vi "WriteData.vi"(6 "TransmissionType":T1, 8 "error in (no error)":errorcluster, 10 "Command":string, 11 "ControlState in":T2 {"ChainMask" format="0x%02x"}) -> (0 "error out":errorcluster, 1 "Data Written?":bool, 2 "return count":u32, 3 "ControlState out":T2 {"ChainMask" format="0x%02x"})   [LabVIEW 2020, in "ArduinoSerialBling.lvlib"]
uses:
  ArduinoSerialBling.lvlib
  ControlState.ctl
  ChainState.ctl
  TransmissionType.ctl
  <vilib>/Instr/_visa.llb/VISA Flush IO Buffer Mask.ctl
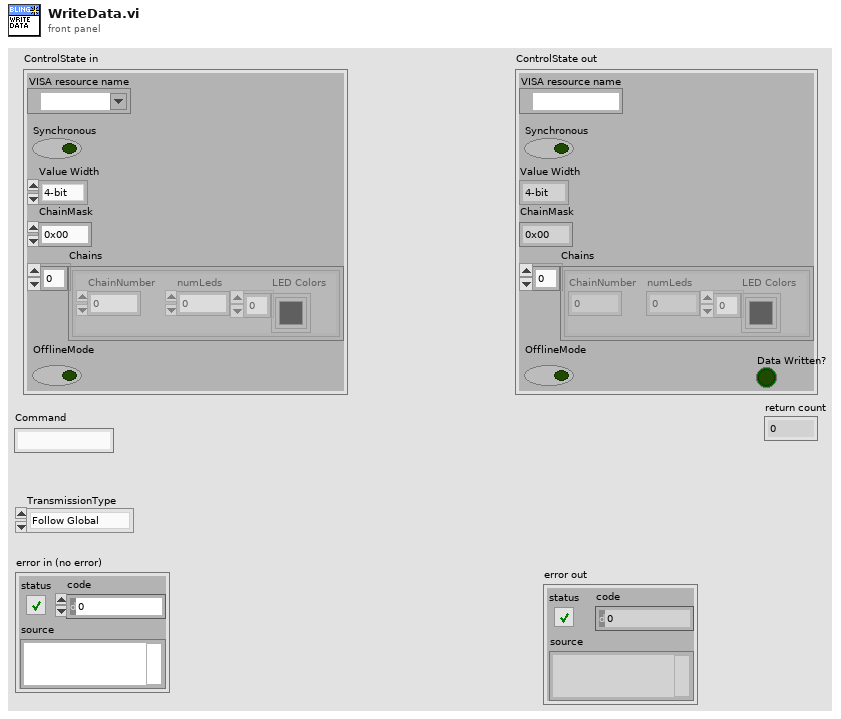
[diagram p1: front panel]
types:
  T1 = typedef "ArduinoSerialBling.lvlib/TransmissionType.ctl" = enum16{"Follow Global", "Asynchronous", "Synchronous"}
  T2 = typedef "ArduinoSerialBling.lvlib/ControlState.ctl" = cluster{"VISA resource name":refnum<visa-resource-name>, "Synchronous":bool, "Value Width":enum16{"4-bit", "8-bit"}, "ChainMask":u8, "Chains":T3[], "OfflineMode":bool}
  T3 = typedef "ArduinoSerialBling.lvlib/ChainState.ctl" = cluster{"ChainNumber":u8, "numLeds":u8, "LED Colors":u32[]}
  T4 = typedef "VISA Flush IO Buffer Mask.ctl" = u16
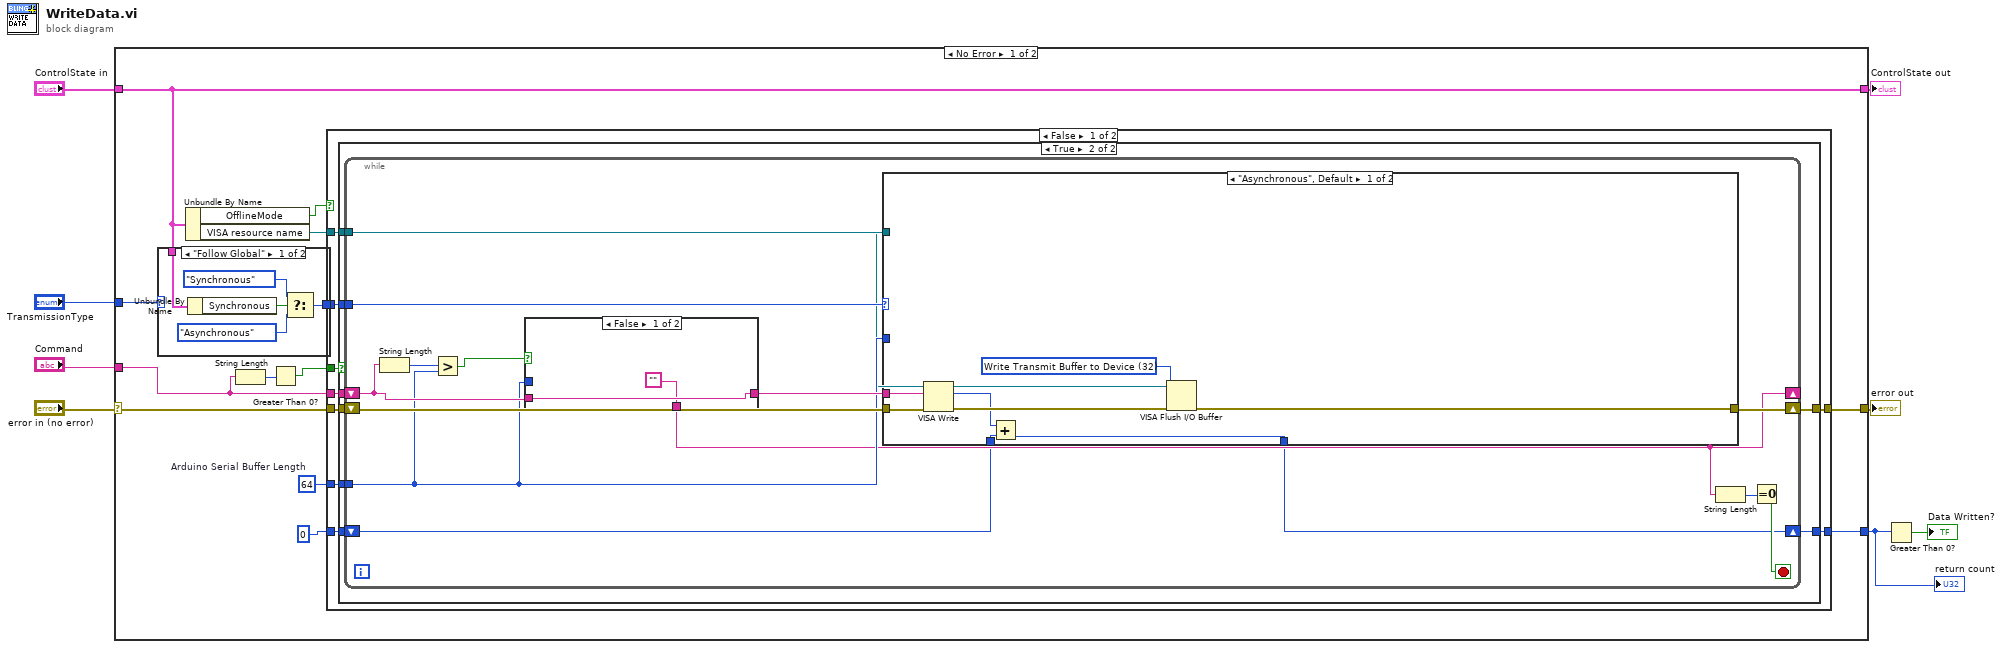
[diagram p0: block diagram]
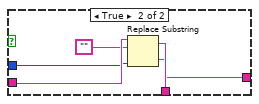
[diagram p3: hidden frame]
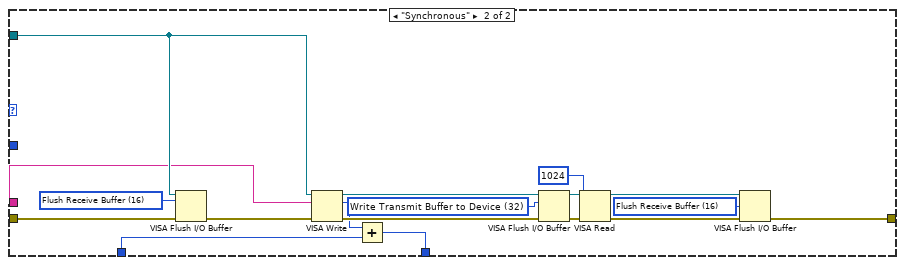
[diagram p4: hidden frame]
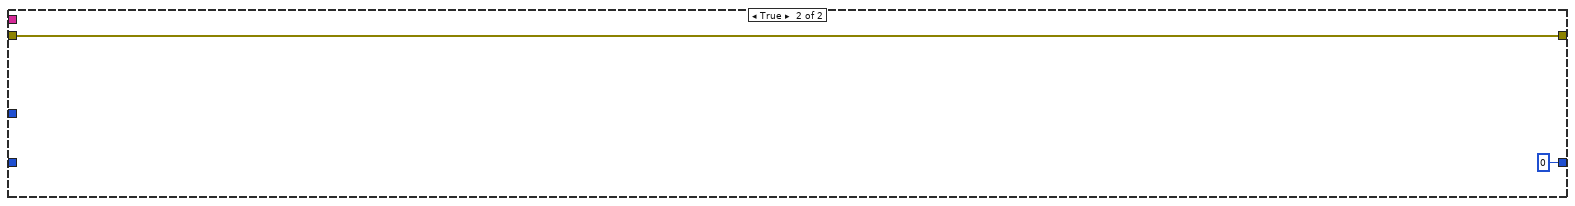
[diagram p5: hidden frame]
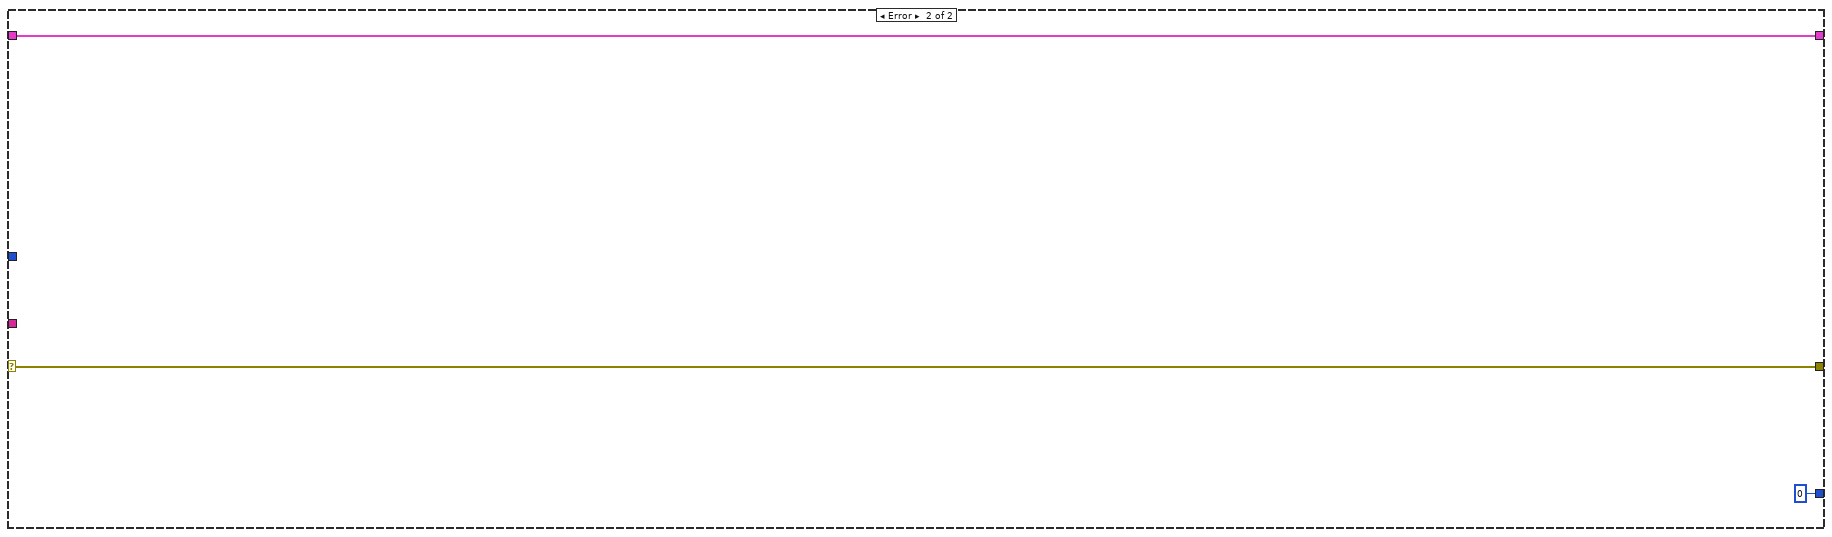
[diagram p7: hidden frame]
diagram:
  n1 = case shown="No Error" "error in (no error)" {
    selector: "error in (no error)" -> [w19 w100]
    tunnel: [w18 w100] -> w7
    tunnel: "ControlState in" -> [w17 w99]
    tunnel: [w17 w99] -> w5
    tunnel: "Command" -> [w13 _]
    tunnel: "TransmissionType" -> [w21 _]
    tunnel: [w10 0] -> w2
    frame No Error {
      w15 = 64  # Arduino Serial Buffer Length
      n2 = case shown="\"Follow Global\"" w21 {
        selector: w21 -> [_ w97]
        tunnel: w17 -> [w96 _]
        tunnel: [w92 w97] -> w20
        frame "Follow Global" {
          n3 = Unbundle By Name(w96) -> ("Synchronous"=w95:bool)
          n4 = Select(t=TransmissionType."Synchronous" ("TransmissionType"), s=w95, f=TransmissionType."Asynchronous") -> (s? t:f=w92:T1)
        }
        frame Default {
        }
      }
      n5 = Unbundle By Name(w17) -> ("OfflineMode"=w9:bool, "VISA resource name"=w16:refnum<visa-resource-name>)
      n6 = String Length(string=w13) -> (length=w12:i32)
      n7 = Greater Than 0?(x=w12) -> (x > 0?=w11:bool)
      n8 = case shown="False" w9 {
        tunnel: w20 -> [w30 _]
        tunnel: w19 -> [w29 w91]
        tunnel: [w28 w91] -> w18
        tunnel: w16 -> [w27 _]
        tunnel: w15 -> [w26 _]
        tunnel: 0 -> [w25 _]
        tunnel: w13 -> [w24 _]
        tunnel: w11 -> [w23 _]
        tunnel: [w22 u32 0] -> w10
        frame False {
          n9 = case shown="True" w23 {
            tunnel: w30 -> [_ w40]
            tunnel: w29 -> [w31 w39]
            tunnel: [w31 w38] -> w28
            tunnel: w27 -> [_ w37]
            tunnel: w26 -> [_ w36]
            tunnel: w24 -> [_ w35]
            tunnel: w25 -> [w32 w34]
            tunnel: [w32 w33] -> w22
            frame False {
            }
            frame True {
              n10 = while {
                tunnel: w40 -> [w54]
                tunnel: w37 -> [w51]
                shift-right: [w52] -> w38
                shift-left: w39 -> [w53]
                shift-right: [w45] -> _
                shift-left: w35 -> [w48]
                tunnel: w36 -> [w46]
                shift-right: [w41] -> w33
                shift-left: w34 -> [w42]
                stop <- w43 stop-if-true
                n11 = String Length(string=w48) -> (length=w50:i32)
                n12 = Greater?(x=w50, y=w46) -> (0:w49:bool)
                n13 = case shown="False" w49 {
                  tunnel: w48 -> [w56 w61]
                  tunnel: w46 -> [_ w60]
                  tunnel: ["" w58] -> w45
                  tunnel: [w56 w57] -> w47
                  frame False {
                  }
                  frame True {
                    n14 = Replace Substring(2:w60, 4:"", 5:w61) -> (0:w57:string, 1:w58:string)  [unwired: 1 in]
                  }
                }
                n15 = case shown="\"Asynchronous\", Default" w54 {
                  tunnel: w53 -> [w71 w87]
                  tunnel: [w66 w89] -> w52
                  tunnel: w51 -> [w70 w86]
                  tunnel: w47 -> [w65 w75]
                  tunnel: w46 -> [_ _]
                  tunnel: w42 -> [w63 w73]
                  tunnel: [w62 w72] -> w41
                  frame "Asynchronous", Default {
                    w67 = T4 32 items=["Flush Receive Buffer"=16, "Write Transmit Buffer to Device"=32, "Flush Receive Buffer (No I/O)"=64, "Flush Transmit Buffer"=128] ("Mask")
                    n16 = VISA Write(VISA resource name=w70, write buffer=w65, error in (no error)=w71) -> (VISA resource name out=w68:refnum<visa-resource-name>, return count=w64:u32, error out=w69:errorcluster)
                    n17 = Add(x=w64, y=w63) -> (x+y=w62:u32)
                    n18 = VISA Flush I/O Buffer(VISA resource name=w68, mask (16)=w67, error in (no error)=w69) -> (error out=w66:errorcluster)  [unwired: 1 out]
                  }
                  frame "Synchronous" {
                    w78 = T4 16 items=["Flush Receive Buffer"=16, "Write Transmit Buffer to Device"=32, "Flush Receive Buffer (No I/O)"=64, "Flush Transmit Buffer"=128] ("Mask")
                    w79 = T4 32 items=["Flush Receive Buffer"=16, "Write Transmit Buffer to Device"=32, "Flush Receive Buffer (No I/O)"=64, "Flush Transmit Buffer"=128] ("Mask")
                    w85 = T4 16 items=["Flush Receive Buffer"=16, "Write Transmit Buffer to Device"=32, "Flush Receive Buffer (No I/O)"=64, "Flush Transmit Buffer"=128] ("Mask")
                    n19 = VISA Flush I/O Buffer(VISA resource name=w86, mask (16)=w85, error in (no error)=w87) -> (error out=w88:errorcluster)  [unwired: 1 out]
                    n20 = VISA Write(VISA resource name=w86, write buffer=w75, error in (no error)=w88) -> (VISA resource name out=w82:refnum<visa-resource-name>, return count=w74:u32, error out=w81:errorcluster)
                    n21 = Add(x=w74, y=w73) -> (x+y=w72:u32)
                    n22 = VISA Flush I/O Buffer(VISA resource name=w82, mask (16)=w79, error in (no error)=w81) -> (VISA resource name out=w83:refnum<visa-resource-name>, error out=w84:errorcluster)
                    n23 = VISA Read(VISA resource name=w83, byte count=u32 1024, error in (no error)=w84) -> (VISA resource name out=w77:refnum<visa-resource-name>, error out=w76:errorcluster)  [unwired: 2 out]
                    n24 = VISA Flush I/O Buffer(VISA resource name=w77, mask (16)=w78, error in (no error)=w76) -> (error out=w89:errorcluster)  [unwired: 1 out]
                  }
                }
                n25 = String Length(string=w45) -> (length=w44:i32)
                n26 = Equal To 0?(x=w44) -> (x = 0?=w43:bool)
              }
            }
          }
        }
        frame True {
        }
      }
    }
    frame Error {
    }
  }
  "ControlState out" <- w5
  "error out" <- w7
  "return count" <- w2
  n27 = Greater Than 0?(x=w2) -> (x > 0?=→"Data Written?":bool)
